vi "insert.vi"(8 "error in (no error)":errorcluster, 10 "To Insert":T1, 11 "Bucket in":refnum<class "Bucket.lvclass">) -> (0 "error out":errorcluster, 3 "Bucket out":refnum<class "Bucket.lvclass">)   [LabVIEW 2017, in "Bucket.lvclass"]
uses:
  <userlib>/836-Library/Data_Structures/Bucket/Bucket.lvclass
  <userlib>/836-Library/Data_Structures/Bucket/Types/KeyValuePair.ctl
  <userlib>/836-Library/Data_Structures/Bucket/Bucket.lvclass/Bucket.ctl
  <vilib>/ErrorRing/Error Ring.xnode
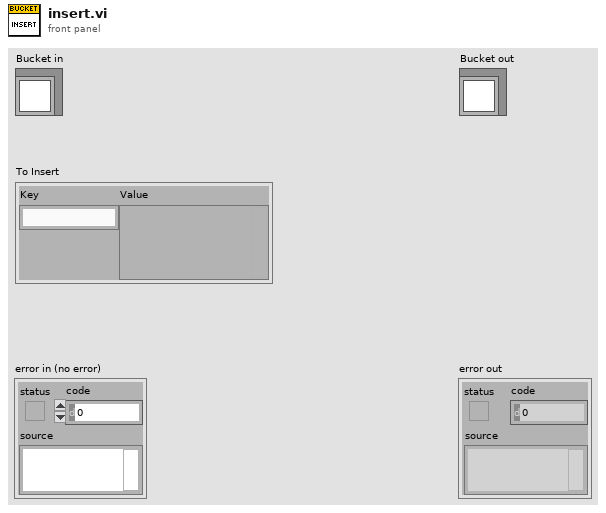
[diagram p1: front panel]
types:
  T1 = typedef "KeyValuePair.ctl" = cluster{"Key":string, "Value":variant}
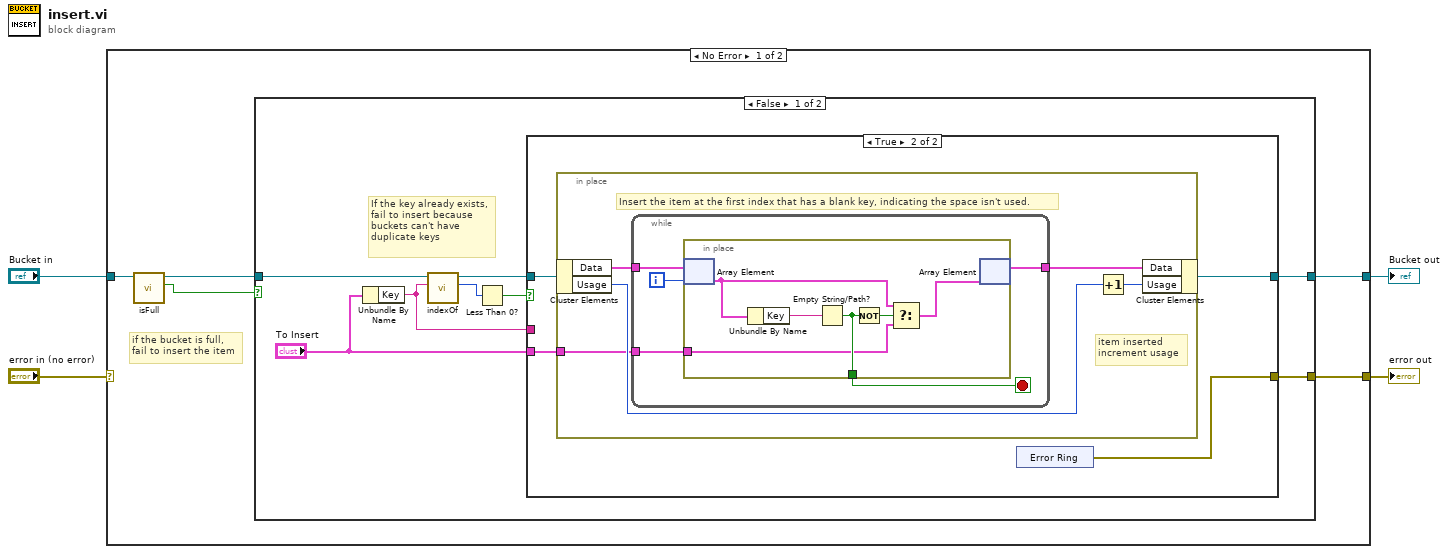
[diagram p0: block diagram]
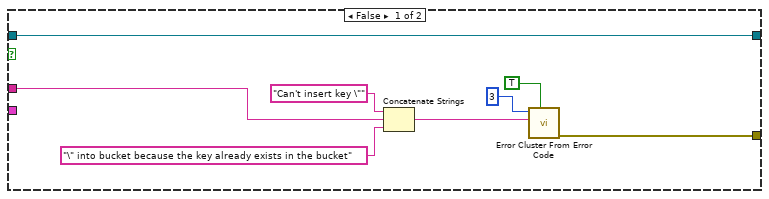
[diagram p2: hidden frame]
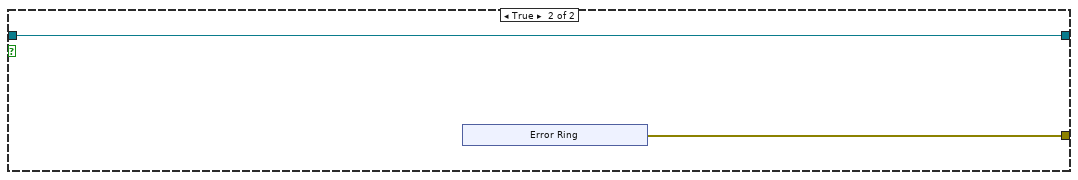
[diagram p3: hidden frame]
diagram:
  n1 = case shown="No Error" "error in (no error)" {
    selector: "error in (no error)" -> [_ w55]
    tunnel: [w5 w55] -> w3
    tunnel: [w6 w54] -> w1
    tunnel: "Bucket in" -> [w9 w54]
    frame No Error {
      # "if the bucket is full,\nfail to insert the item"
      n2 = call <userlib>:"isFull.vi"("Bucket in"=w9) -> ("Full?"=w8:bool, "Bucket out"=w7:refnum<class "Bucket.lvclass">)  [unwired: 8 in, 1 out]
      n3 = case shown="False" w8 {
        tunnel: [w16 w48] -> w5
        tunnel: w7 -> [w14 w47]
        tunnel: [w17 w47] -> w6
        frame False {
          # "If the key already exists,\nfail to insert because\nbuckets can't have\nduplicate keys"
          n4 = Unbundle By Name("To Insert") -> ("Key"=w10:string)
          n5 = call <userlib>:"indexOf.vi"("Key"=w10, "Bucket in"=w14) -> ("Index"=w12:i32, "Bucket out"=w13:refnum<class "Bucket.lvclass">)  [unwired: 7 in, 1 out]
          n6 = Less Than 0?(x=w12) -> (x < 0?=w11:bool)
          n7 = case shown="True" w11 {
            tunnel: [w25 w29] -> w17
            tunnel: [w18 w28] -> w16
            tunnel: "To Insert" -> [_ w27]
            tunnel: w13 -> [w25 w26]
            tunnel: w10 -> [w21 _]
            frame False {
              n8 = Concatenate Strings("Can't insert key \"" ("string"), w21, "\" into bucket because the key already exists in the bucket" ("string")) -> (w22:string)
              n9 = call <vilib>:"Error Cluster From Error Code.vi"("show call chain? (False)"=TRUE, "error message (\"\")"=w22, "error code (0)"=3) -> ("error out"=w18:errorcluster)  [unwired: 6 in]
            }
            frame True {
              n10 = in-place {
                in-place-border: w27 -> [w31]
                # "item inserted\nincrement usage"
                # "Insert the item at the first index that has a blank key, indicating the space isn't used."
                n11 = in-place-cluster #1(w26) -> ("Data"=w35:T1[], "Usage"=w32:u32)
                n12 = while {
                  tunnel: w35 -> [w40]
                  tunnel: [w37] -> w34
                  tunnel: w31 -> [w36]
                  i -> [w39]
                  stop <- w38 stop-if-true
                  n13 = in-place {
                    in-place-border: [w42] -> w38
                    in-place-border: w36 -> [w41]
                    n14 = in-place-array #2(w40, w39) -> (w44:T1)
                    n15 = Unbundle By Name(w44) -> ("Key"=w46:string)
                    n16 = Empty String/Path?(string/path=w46) -> (empty?=w42:bool)
                    n17 = Not(x=w42) -> (.not. x?=w45:bool)
                    n18 = Select(t=w44, s=w45, f=w41) -> (s? t:f=w43:T1)
                    n19 = in-place-array #2(w43) -> (w37:T1[])  [unwired: 1 out]
                  }
                }
                n20 = Increment(x=w32) -> (x+1=w33:u32)
                n21 = in-place-cluster #1("Data"=w34, "Usage"=w33) -> (w29:refnum<class "Bucket.lvclass">)
              }
              n22 = xnode "Error Ring"() -> ("error out"=w28:errorcluster)
            }
          }
        }
        frame True {
          n23 = xnode "Error Ring"() -> ("error out"=w48:errorcluster)
        }
      }
    }
    frame Error {
    }
  }
  "error out" <- w3
  "Bucket out" <- w1
